vi "Set_Control_Relays.vi"(8 "error in (no error)":errorcluster caption="entrée d'erreur (pas d'erreur)", 10 "Tab_Num_Relay":u8[](array[numeric]), 11 "Class Relay_Board (Default) en entrée":refnum<class "Class Relay_Board (Default).lvclass">) -> (0 "error out":errorcluster caption="sortie d'erreur", 3 "Class Relay_Board (Default) en sortie":refnum<class "Class Relay_Board (Default).lvclass">)   [LabVIEW 2020, in "Library Instrument & Equipement.lvlib" / "Library Relay_Board.lvlib" / "Class Relay_Board (Default).lvclass"]
uses:
  Class Relay_Board (Default).lvclass
  Class Relay_Board (Default).lvclass/Class Relay_Board (Default).ctl
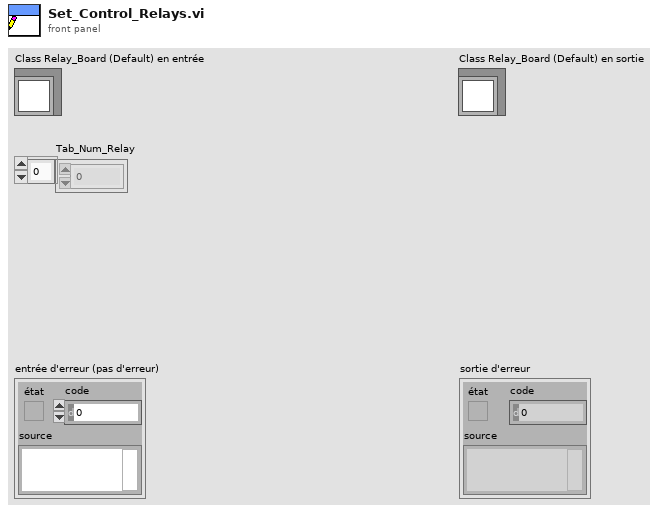
[diagram p1: front panel]
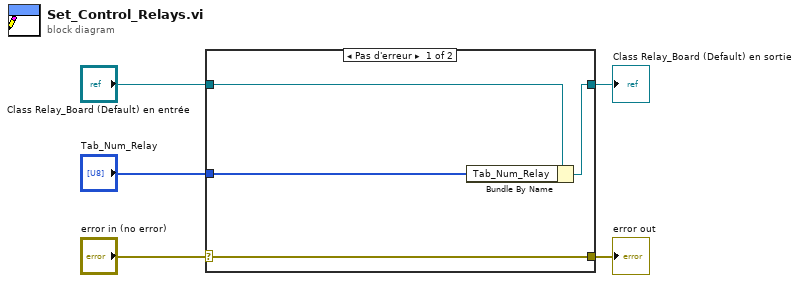
[diagram p0: block diagram]
diagram:
  n1 = case shown="Pas d'erreur" "error in (no error)" {
    selector: "error in (no error)" -> [w9 w10]
    tunnel: [w9 w10] -> w4
    tunnel: [w7 w11] -> w2
    tunnel: "Class Relay_Board (Default) en entrée" -> [w8 w11]
    tunnel: "Tab_Num_Relay" -> [w6 _]
    frame No Error {
      n2 = Bundle By Name(cluster=w8, "Tab_Num_Relay"=w6) -> (w7:refnum<class "Class Relay_Board (Default).lvclass">)
    }
    frame Error {
    }
  }
  "error out" <- w4
  "Class Relay_Board (Default) en sortie" <- w2
